vi "String Included.vi"() -> ()   [LabVIEW 2017, in "Transparent Assertions.Tests.lvlib" / "Assert String Not Contains String Ignoring Case.lvlib"]
uses:
  Assert String Not Contains String Ignoring Case.lvlib
  src/Transparent Assertions/Transparent Assertions.lvlib
panel:
  out "error out":errorcluster
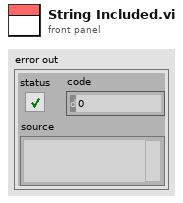
[diagram p1: front panel]
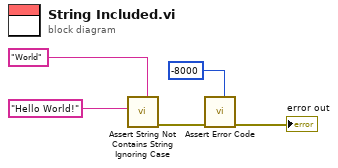
[diagram p0: block diagram]
diagram:
  n1 = call "Assert String Not Contains String Ignoring Case.vi"("Needle"="World", "Haystack"="Hello World!") -> ("error out"=w3:errorcluster)  [unwired: 9 in]
  n2 = call "Assert Error Code.vi"("Expected"=-8000, "error in (no error)"=w3) -> ("error out"=→"error out":errorcluster)  [unwired: 9 in]
